vi "AFG3352X.enable output.vi"(0 "i ref in":refnum<vi>, 1 "Channel (1: 1)":u16(ring)=1 items=["1"=1, "2"=2], 2 "outputEnable":bool, 3 "ms timeout (10000)":i32=10000, 5 "error in (no error)":errorcluster) -> (14 "i ref out":refnum<vi>, 17 "timed out":bool, 19 "error out":errorcluster)   [LabVIEW 2014, in "AFG3352X.lvlib"]
doc: "Enables the output of the device."
uses:
  AFG3352X.lvlib
  CS_Core/CSApplicationBaseClasses/AFGBase/AFGBase.serviceType.ctl
  CS_Core/CSApplicationBaseClasses/AFGBase/AFGBase.directionType.ctl
  CSlibraries/UtilityLib/UtilityLib.valueStatus.ctl
  CS_Core/CSApplicationBaseClasses/DeviceBase/DeviceBase.lvlib
  CS_Core/CSApplicationBaseClasses/AFGBase/AFGBase.lvlib
  CSlibraries/UtilityLib/UtilityLib.lvlib
  instr.lib/Agilent 3352X Series/Agilent 3352X Series.lvlib
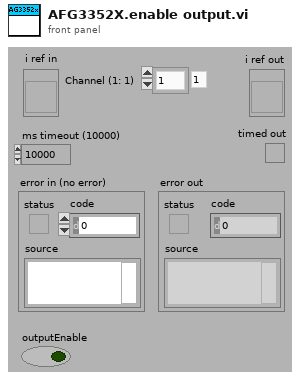
[diagram p1: front panel]
types:
  T1 = typedef "UtilityLib.lvlib/UtilityLib.valueStatus.ctl" = enum16{"no info available", "stand by/off", "on", "warning", "alarm/malfunction", "not implemented", "user action required", "important information", "system default", "control default", "indicator default", "button default"}
  T2 = typedef "AFGBase.lvlib/AFGBase.directionType.ctl" = enum16{"unknown", "update actual value", "update nominal value", "update both"}
  T3 = typedef "AFGBase.lvlib/AFGBase.serviceType.ctl" = enum16{"frequency", "amplitude", "phase", "DCOffset", "enableOutput", "trigger", "waveformType"}
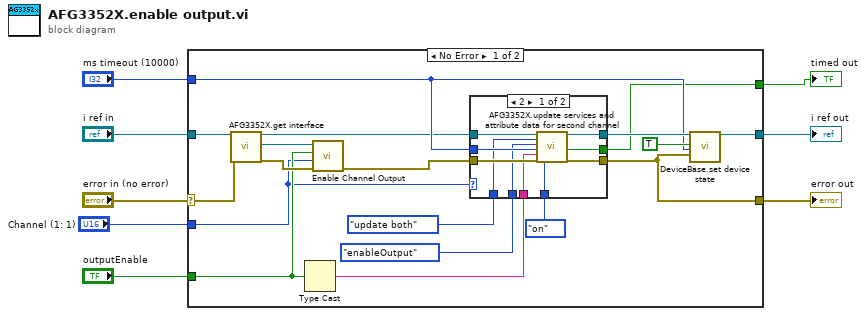
[diagram p0: block diagram]
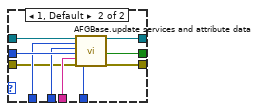
[diagram p2: hidden frame]
diagram:
  n1 = case shown="No Error" "error in (no error)" {
    selector: "error in (no error)" -> [w16 w47]
    tunnel: [w26 w48] -> w8
    tunnel: "ms timeout (10000)" -> [w22 _]
    tunnel: "i ref in" -> [w17 w48]
    tunnel: [w23 w47] -> w4
    tunnel: "outputEnable" -> [w12 _]
    tunnel: [w10 _] -> w2
    tunnel: "Channel (1: 1)" -> [w9 _]
    frame No Error {
      n2 = call "AFG3352X.get interface.vi"("i ref in"=w17, "error in (no error)"=w16) -> ("i ref out"=w15:refnum<vi>, "interface"=w13:refnum<visa-resource-name>, "error out"=w14:errorcluster)  [unwired: 15 in]
      n3 = Type Cast(x=w12) -> (*(type *) &x=w20:string)  [unwired: 1 in]
      n4 = call "Enable Channel Output.vi"("error in (no error)"=w14, "Channel (1: 1)"=w9, "Enable Output (T: Enable)"=w12, "VISA resource name"=w13) -> ("error out"=w11:errorcluster)  [unwired: 6 in, 1 out]
      n5 = case shown="2" w9 {
        tunnel: [w35 w46] -> w24
        tunnel: [w34 w45] -> w23
        tunnel: w22 -> [w29 w44]
        tunnel: AFGBase.serviceType."enableOutput" ("service") -> [w28 w43]
        tunnel: w20 -> [w30 w42]
        tunnel: AFGBase.directionType."update both" ("direction") -> [w27 w41]
        tunnel: UtilityLib.valueStatus."on" ("quality") -> [w31 w40]
        tunnel: w15 -> [w36 w39]
        tunnel: w11 -> [w32 w38]
        tunnel: [w33 w37] -> w10
        frame 2 {
          n6 = call "AFG3352X.update services and attribute data for second channel.vi"("i ref in"=w36, "direction"=w27, "service"=w28, "ms timeout (10000)"=w29, "value"=w30, "error in (no error)"=w32, "quality"=w31) -> ("i ref out"=w35:refnum<vi>, "timed out"=w33:bool, "error out"=w34:errorcluster)  [unwired: 10 in]
        }
        frame 1, Default {
          n7 = call "AFGBase.update services and attribute data.vi"("i ref in"=w39, "direction"=w41, "service"=w43, "ms timeout (10000)"=w44, "value"=w42, "error in (no error)"=w38, "quality"=w40) -> ("i ref out"=w46:refnum<vi>, "timed out"=w37:bool, "error out"=w45:errorcluster)  [unwired: 10 in]
        }
      }
      n8 = call "DeviceBase.set device state.vi"("i ref in"=w24, "implicit"=TRUE, "ms timeout (10000)"=w22, "device error"=w23) -> ("i ref out"=w26:refnum<vi>)  [unwired: 13 in, 2 out]
    }
    frame Error {
    }
  }
  "error out" <- w4
  "i ref out" <- w8
  "timed out" <- w2
